vi "RemanentMagnetization.vi"(8 "B":dbl[](array[numeric]), 11 "H":dbl[](array[numeric])) -> (2 "Rem Mag":dbl)   [LabVIEW 2019]
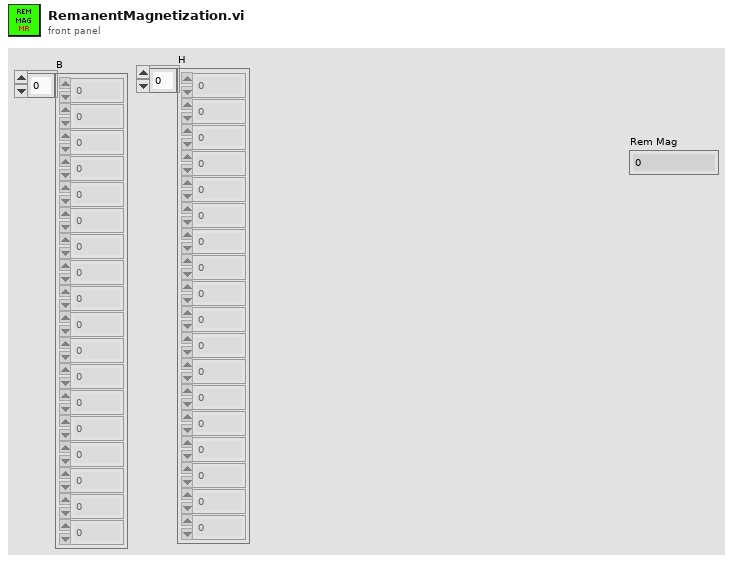
[diagram p1: front panel]
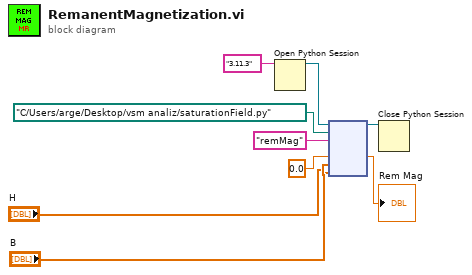
[diagram p0: block diagram]
diagram:
  n1 = Open Python Session(python version="3.11.3" ("Python version")) -> (session out=w8:refnum<k35>)  [unwired: 2 in, 1 out]
  n2 = node(w8, path "C:/Users/arge/Desktop/vsm analiz/saturationField.py" ("module path"), "remMag" ("function name"), 0.0, "B", "H") -> (w3:refnum<k35>, →"Rem Mag":dbl)  [unwired: 3 in, 3 out]
  n3 = Close Python Session(session in=w3) -> ()  [unwired: 1 in, 1 out]
